vi "Module Running as Singleton--error.vi"() -> (0 "error out":errorcluster)   [LabVIEW 2025, in "Data Log.lvlib"]
doc: "Outputs an error cluster containing a custom error code indicating the module was running as a singleton, but Start Module has the 'Run as Singleton' input set to FALSE.\n_____\nBased on DQMH Dev Tools: Project Template 7.1.2.1547."
uses:
  Data Log.lvlib
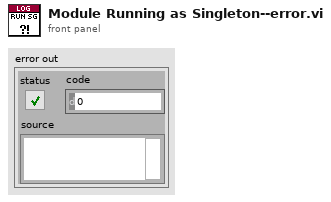
[diagram p1: front panel]
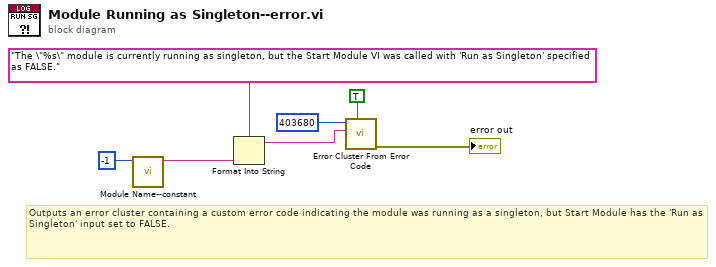
[diagram p0: block diagram]
diagram:
  # "Outputs an error cluster containing a custom error code indicating the module was running as a singleton, but Start Module has the 'Run as Singleton' input set to FALSE."
  n1 = call "Module Name--constant.vi"("Module ID"=-1) -> ("Module Name"=w2:string)  [unwired: 10 in]
  n2 = Format Into String(format string="The \"%s\" module is currently running as singleton, but the Start Module VI was called with 'Run as Singleton' specified as FALSE.", w2) -> (resulting string=w6:string)  [unwired: 2 in, 1 out]
  n3 = call <vilib>:"Error Cluster From Error Code.vi"("show call chain? (False)"=TRUE, "error message (\"\")"=w6, "error code (0)"=403680) -> ("error out"=→"error out":errorcluster)  [unwired: 6 in]
